vi "DestroySelfReference.vi"(8 "error in (no error)":errorcluster, 11 "GUI":refnum<class "GUI.lvclass">) -> (0 "error out":errorcluster, 3 "GUI out":refnum<class "GUI.lvclass">)   [LabVIEW 2022 SP3, in "GUI.lvclass"]
doc: "JKI State Machine Objects (SMO) 1.0.0.5\nJKI - JKI\nCopyright (c) 2016, JKI"
uses:
  GUI.lvclass
  GUI.lvclass/GUI.ctl
  <vilib>/JKI/JKI SMO/SMO/SMO.lvclass
panel:
  # "For instructions on how to use the JKI State Machine Objects, examples and video tutorials, visit:\nhttp://jki.net/state-machine-objects/\n\nJKI State Machine Objects™\nhttp://jki.net/state-machine-objects/\nCopyright (C) 2005-2015, JKI <info@jki.net>\nALL RIGHTS RESERVED"
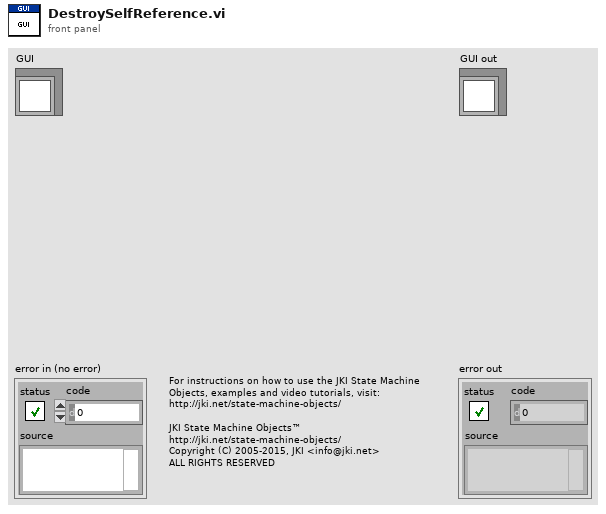
[diagram p1: front panel]
types:
  T1 = typedef "GUI.lvclass/PrivateData--Ref.ctl" = refnum<data-value>
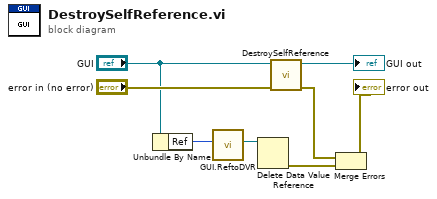
[diagram p0: block diagram]
diagram:
  n1 = Unbundle By Name("GUI") -> ("Ref"=w2:u32)
  n2 = call "GUI.ReftoDVR.vi"("Ref"=w2) -> ("Ref"=w1:T1)  [unwired: 10 in]
  n3 = Delete Data Value Reference(data value reference=w1) -> (error out=w5:errorcluster)  [unwired: 1 in, 1 out]
  n4 = call-parent "DestroySelfReference.vi"("error in (no error)"="error in (no error)", "SMO"="GUI") -> ("error out"=w4:errorcluster, "SMO out"=→"GUI out":refnum<class "GUI.lvclass">)  [unwired: 8 in]
  n5 = Merge Errors(w4, w5) -> (→"error out":errorcluster)
